vi "DHE_set_custom.vi"(0 "fd":i32, 7 "args":string, 11 "error in (no error)":errorcluster) -> (4 "fd out":i32, 8 "str result":string, 15 "error out":errorcluster)   [LabVIEW 2016]
doc: "This VI closes the I/O interface with the instrument."
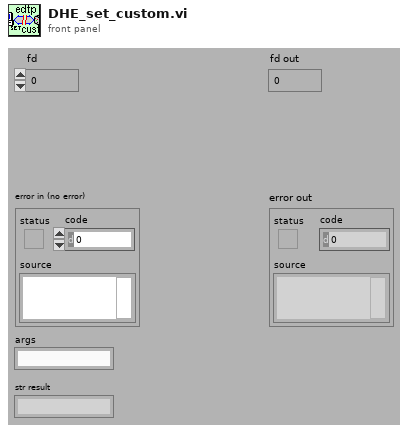
[diagram p1: front panel]
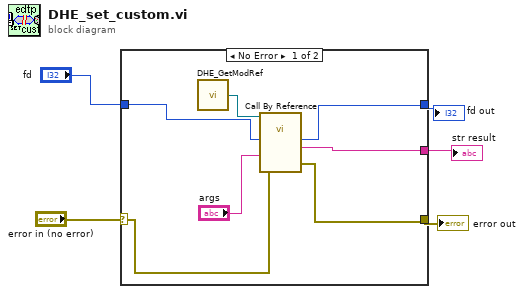
[diagram p0: block diagram]
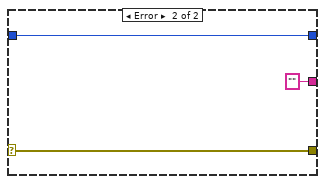
[diagram p2: hidden frame]
diagram:
  n1 = case shown="No Error" "error in (no error)" {
    selector: "error in (no error)" -> [w8 w14]
    tunnel: "fd" -> [w9 w15]
    tunnel: [w11 w14] -> w4
    tunnel: [w10 w15] -> w3
    tunnel: [w6 "" ("str result")] -> w1
    frame No Error {
      n2 = call "DHE_GetModRef.vi"() -> ("DHE_ModRef"=w12:refnum<vi>)  [unwired: 9 out]
      n3 = call-by-ref "?"(reference=w12, "error in (no error)"=w8, "arguments"="args", "fd in"=w9) -> ("error out"=w11:errorcluster, "str result"=w6:string, "fd out"=w10:i32)  [unwired: 6 in, 3 out]
    }
    frame Error {
    }
  }
  "error out" <- w4
  "fd out" <- w3
  "str result" <- w1
